vi "Process.WaitonStart.vi"(8 "error in (no error)":errorcluster, 11 "Process in":refnum<class "Process.lvclass">) -> (0 "error out":errorcluster, 2 "notification":bool, 3 "Process out":refnum<class "Process.lvclass">)   [LabVIEW 2015, in "VS Inline Async API.lvlib" / "Process.lvclass"]
uses:
  Process.lvclass
  Process.lvclass/Process.ctl
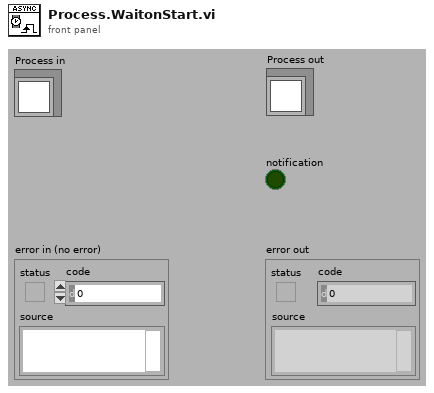
[diagram p1: front panel]
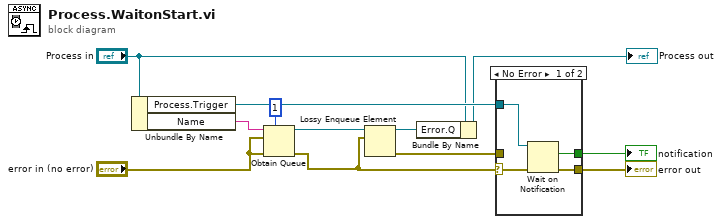
[diagram p0: block diagram]
diagram:
  n1 = Unbundle By Name("Process in") -> ("Process.Trigger"=w4:refnum<notifier>, "Name"=w7:string)
  n2 = Obtain Queue(max queue size (-1, unlimited)=1, name (unnamed)=w7, element data type="error in (no error)", error in (no error)="error in (no error)") -> (queue out=w6:refnum<queue>, error out=w8:errorcluster)  [unwired: 1 in, 1 out]
  n3 = Lossy Enqueue Element(queue=w6, element=w8) -> (queue out=w5:refnum<queue>, error out=w10:errorcluster)  [unwired: 1 in, 2 out]
  n4 = Bundle By Name(cluster="Process in", "Error.Q"=w5) -> (→"Process out":refnum<class "Process.lvclass">)
  n5 = case shown="No Error" w8 {
    selector: w8 -> [w14 w17]
    tunnel: [w16 w17] -> w12
    tunnel: [w15 _] -> w11
    tunnel: w10 -> [_ _]
    tunnel: w4 -> [w13 _]
    frame No Error {
      n6 = Wait on Notification(notifier=w13, error in (no error)=w14) -> (notification=w15:bool, error out=w16:errorcluster)  [unwired: 2 in, 2 out]
    }
    frame Error {
    }
  }
  "error out" <- w12
  "notification" <- w11
